vi "(ball) Compare (SubVI).vi"(6 "Boolean":bool, 7 "Balls to remember":i32, 9 "Ball number":i32, 10 "Color classes":i32[](array[numeric]), 11 "Boolean in":refnum<vi>) -> (3 "ball match":bool)   [LabVIEW 2017]
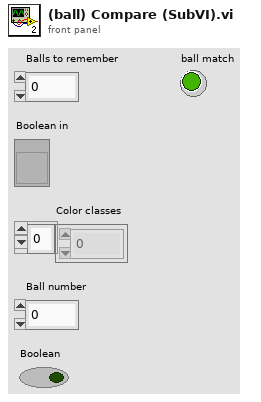
[diagram p1: front panel]
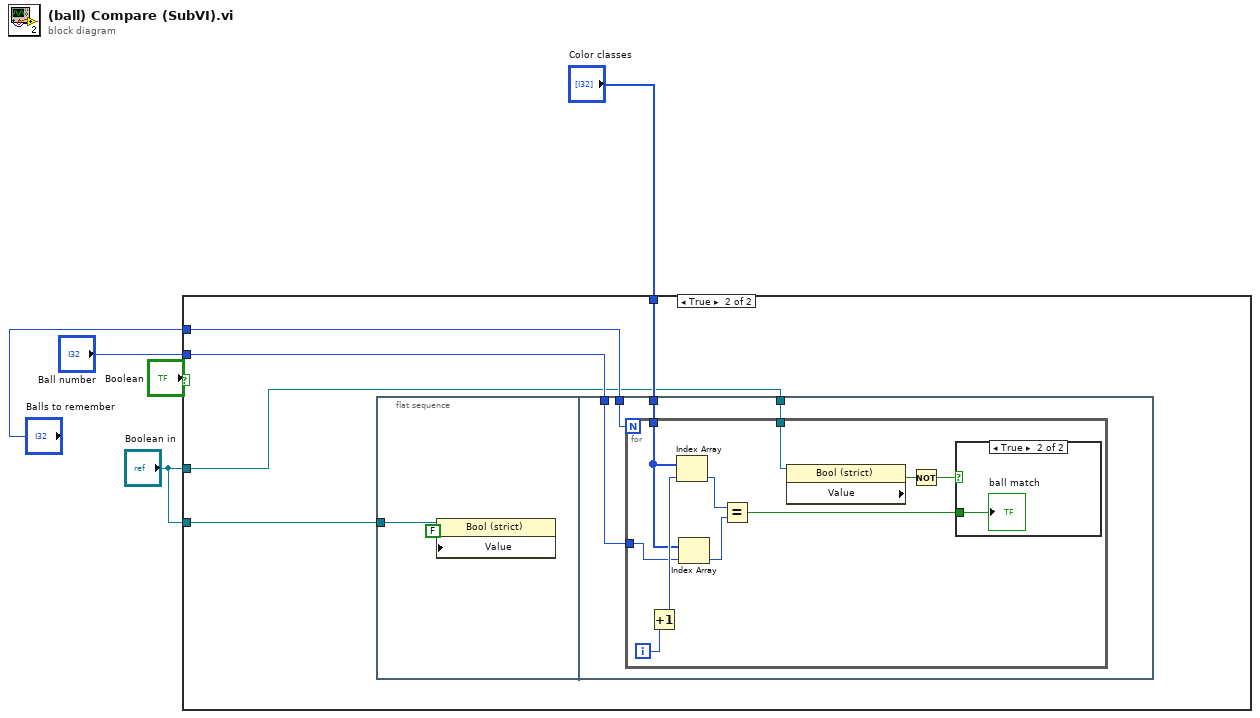
[diagram p0: block diagram]
diagram:
  n1 = case shown="True" "Boolean" {
    tunnel: "Balls to remember" -> [_ w10]
    tunnel: "Ball number" -> [_ w9]
    tunnel: "Color classes" -> [_ w8]
    tunnel: "Boolean in" -> [_ w7]
    tunnel: "Boolean in" -> [_ w6]
    frame False {
    }
    frame True {
      n2 = flat-sequence {
        tunnel: w6 -> [w11]
        tunnel: w10 -> [w16]
        tunnel: w9 -> [w15]
        tunnel: w8 -> [w14]
        tunnel: w7 -> [w13]
        frame #0 {
          n3 = property class="Bool (strict)"(reference=w11, "Value"=FALSE ("ball match")) -> ()  [unwired: 1 in, 2 out]
        }
        frame #1 {
          n4 = for {
            N: w16 -> [_]
            tunnel: w15 -> [w20]
            tunnel: w14 -> [w18]
            tunnel: w13 -> [w17]
            i -> [w22]
            n5 = Increment(x=w22) -> (x+1=w21:i32)
            n6 = Index Array(array=w18, index=w21) -> (element=w24:i32)
            n7 = Index Array(array=w18, index=w20) -> (element=w23:i32)
            n8 = Equal?(x=w24, y=w23) -> (x = y?=w25:bool)
            n9 = property class="Bool (strict)"(reference=w17) -> ("Value"=w19:bool)  [unwired: 1 in, 2 out]
            n10 = Not(x=w19) -> (.not. x?=w26:bool)
            n11 = case shown="True" w26 {
              tunnel: w25 -> [_ w27]
              frame False {
              }
              frame True {
                "ball match" <- w27
              }
            }
          }
        }
      }
    }
  }
